vi "Append Horizontal Line to Report.vi"(0 "report in":refnum<class "NI_Word.lvclass">, 1 "size (default)":i32=1, 2 "MS Office parameters":T2, 5 "align (default)":T1, 9 "width (100=default)":dbl=100.0 format="%.2f", 11 "error in (no error)":errorcluster, 12 "width units":enum16{"Pixels", "Percentage"}(ring)=enum."Percentage", 13 "noshade (F)":bool) -> (4 "report out":refnum<class "NI_Word.lvclass">, 15 "error out":errorcluster)   [LabVIEW 2023, in "NI_Word.lvclass"]
doc: "Creates a horizontal rule in an HTML, Word, or Excel report. You cannot use this VI with standard reports."
uses:
  NI_Word.lvclass
  <vilib>/Utility/NIReport.llb/HTML Report Text Alignment.ctl
  <vilib>/Utility/NIReport.llb/NI_ReportGenerationCore.lvlib
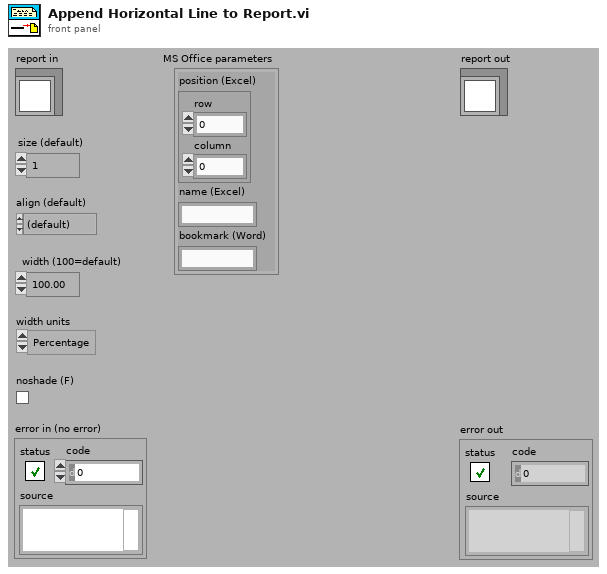
[diagram p1: front panel]
types:
  T1 = typedef "NI_ReportGenerationCore.lvlib/HTML Report Text Alignment.ctl" = enum16{"(default)", "LEFT", "CENTER", "RIGHT"}
  T2 = cluster{"position (Excel)":cluster{"row":i32, "column":i32}, "name (Excel)":string, "bookmark (Word)":string}
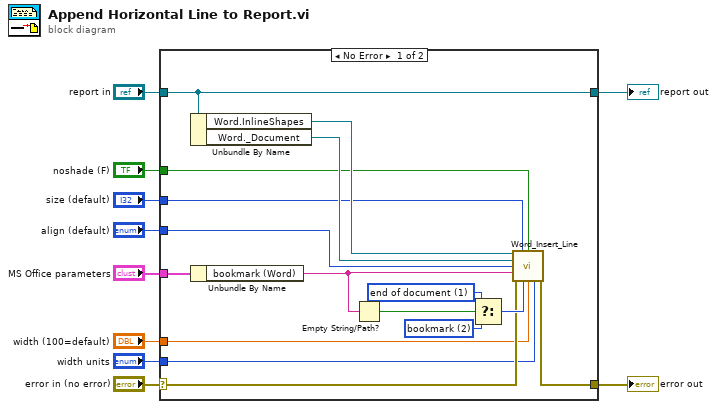
[diagram p0: block diagram]
diagram:
  n1 = case shown="No Error" "error in (no error)" {
    selector: "error in (no error)" -> [w18 w28]
    tunnel: [w17 w28] -> w9
    tunnel: [w19 w27] -> w7
    tunnel: "report in" -> [w19 w27]
    tunnel: "noshade (F)" -> [w16 _]
    tunnel: "align (default)" -> [w15 _]
    tunnel: "size (default)" -> [w14 _]
    tunnel: "MS Office parameters" -> [w13 _]
    tunnel: "width (100=default)" -> [w12 _]
    tunnel: "width units" -> [w11 _]
    frame No Error {
      w20 = u16 2 items=["begining of document", "end of document", "bookmark", "custom"] ("Insertion point")
      w21 = u16 1 items=["begining of document", "end of document", "bookmark", "custom"] ("Insertion point")
      n2 = Unbundle By Name(w19) -> ("Word.InlineShapes"=w24:refnum<k7>, "Word._Document"=w25:refnum<k7>)
      n3 = Unbundle By Name(w13) -> ("bookmark (Word)"=w26:string)
      n4 = Empty String/Path?(string/path=w26) -> (empty?=w22:bool)
      n5 = Select(t=w21, s=w22, f=w20) -> (s? t:f=w23:u16)
      n6 = call <vilib>:"Word_Insert_Line.vi"("Word.InlineShapes"=w24, "size (default)"=w14, "noshade (F)"=w16, "Word._Document"=w25, "align (default)"=w15, "bookmark (Word)"=w26, "error in"=w18, "Insertion point"=w23, "width (0=default)"=w12, "width units"=w11) -> ("error out"=w17:errorcluster)  [unwired: 5 out]
    }
    frame Error {
    }
  }
  "error out" <- w9
  "report out" <- w7
